vi "WFDC Scan Focus.vi"(0 "Ref Image":T1, 5 "Camera Notifier":string, 7 "Z Stage Notifier":string, 9 "No. of Steps":i32=40, 11 "Step Size (µm)":dbl=1.0) -> (4 "Z Stage Notifier (Dup)":string, 8 "Pos vs. Corr":dbl[][](array[numeric]), 15 "Canceled?":bool)   [LabVIEW 2020]
uses:
  <vilib>/vision/Image Controls.llb/IMAQ Image.ctl
  <vilib>/Utility/miscctls.llb/LVPointTypeDef.ctl
  Device Library/Stages/Stages Controls/Stage Actions.ctl
panel:
  in  "Cancel":bool
  out "Position vs. Normalized Correlation":cluster{dbl[], dbl[]}(graph)
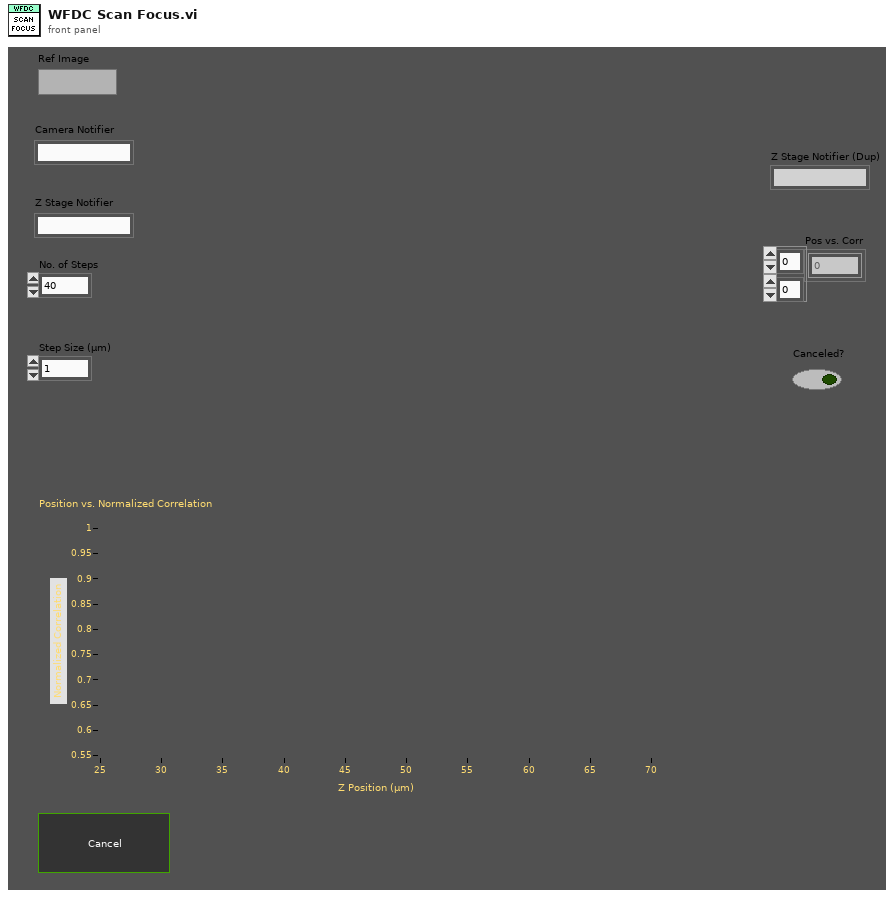
[diagram p1: front panel]
types:
  T1 = typedef "IMAQ Image.ctl" = refnum<image>
  T2 = enum16{"Always On", "Always Off", "Off While Running"}
  T3 = typedef "LVPointTypeDef.ctl" = cluster{"Horizontal":i16, "Vertical":i16}
  T4 = typedef "LVRectTypeDef.ctl" = cluster{"Left":i16, "Top":i16, "Right":i16, "Bottom":i16}
  T5 = typedef "LVBoundsTypeDef.ctl" = cluster{"Width":u32, "Height":u32}
  T6 = typedef "Stage Actions.ctl" = enum16{"Get Position", "MVR", "MOVE", "HALT", "ONTARGET", "ERROR", "REFERENCE", "INIT", "VELOCITY", "STATUS", "EXIT", "HOME", "ZEROPOS", "NANOPOS", "ANALOG", "QUIT"}
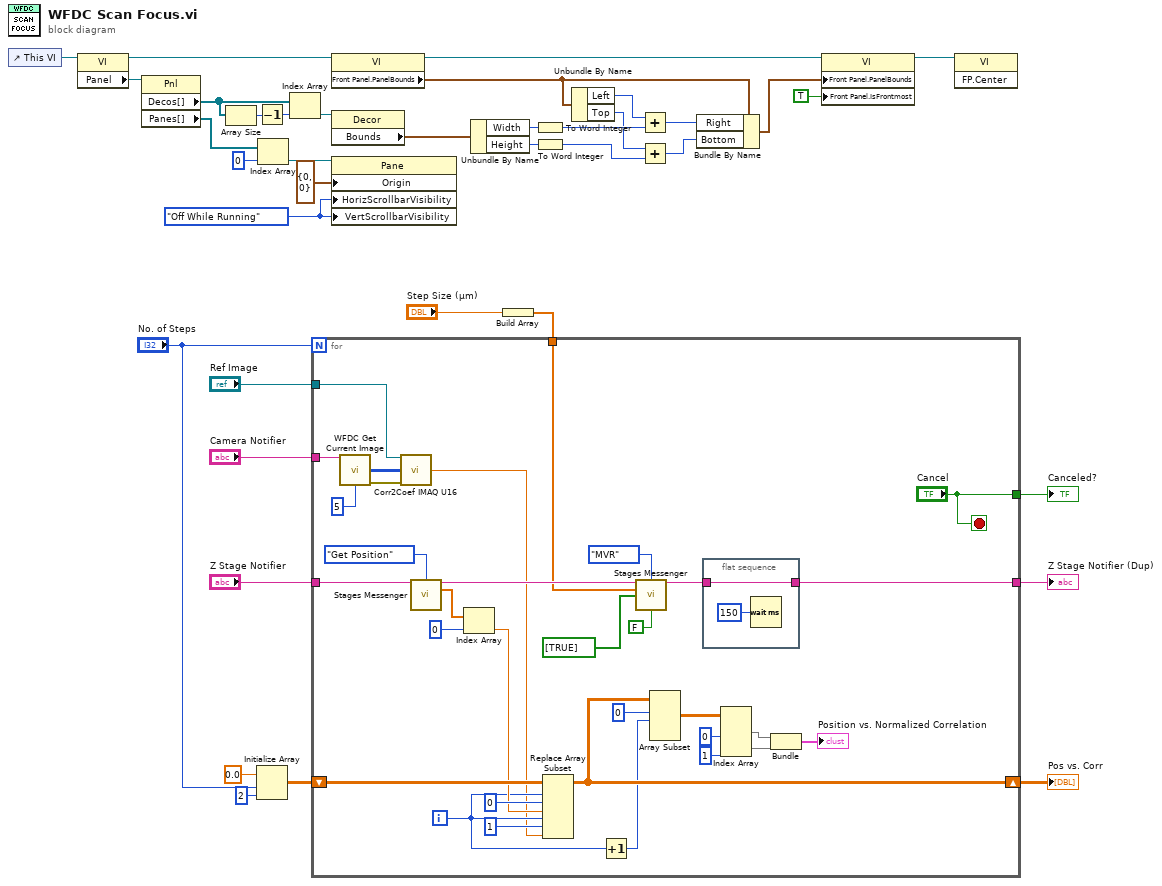
[diagram p0: block diagram]
diagram:
  w16 = T2."Off While Running" ("Vertical Scrollbar Visibility")
  n1 = control-ref of="This VI"() -> (w3:refnum<vi>)
  n2 = property class="VI"(reference=w3) -> (reference out=w17:refnum<vi>, "Panel"=w10:refnum<vi>)  [unwired: 1 in, 1 out]
  n3 = property class="Pnl"(reference=w10) -> ("Decos[]"=w9:refnum<vi>[], "Panes[]"=w13:refnum<vi>[])  [unwired: 1 in, 2 out]
  n4 = Array Size(array=w9) -> (size(s)=w7:i32)
  n5 = Decrement(x=w7) -> (x-1=w8:i32)
  n6 = Initialize Array(0.0 ("element"), "No. of Steps", 2 ("dimension size")) -> (w37:dbl[][])
  n7 = Index Array(array=w13, index=0) -> (element=w12:refnum<vi>)
  n8 = Index Array(array=w9, index=w8) -> (element=w15:refnum<vi>)
  n9 = property class="VI"(reference=w17) -> (reference out=w19:refnum<vi>, "Front Panel.PanelBounds"=w20:T4)  [unwired: 1 in, 1 out]
  n10 = property class="Decor"(reference=w15) -> ("Bounds"=w18:T5)  [unwired: 1 in, 2 out]
  n11 = property class="Pane"(reference=w12, "Origin"=T3 {"Horizontal"=0, "Vertical"=0}, "HorizScrollbarVisibility"=w16, "VertScrollbarVisibility"=w16) -> ()  [unwired: 1 in, 2 out]
  n12 = Unbundle By Name(w18) -> ("Width"=w23:u32, "Height"=w26:u32)
  n13 = Build Array("Step Size (µm)") -> (w29:dbl[])
  n14 = for {
    N: "No. of Steps" -> [_]
    tunnel: "Camera Notifier" -> [w69]
    tunnel: "Z Stage Notifier" -> [w65]
    tunnel: "Ref Image" -> [w40]
    shift-right: [w52] -> w31
    shift-left: w37 -> [w62]
    tunnel: [w43] -> w34
    tunnel: w29 -> [w47]
    tunnel: ["Cancel"] -> w28
    i -> [w49]
    stop <- "Cancel" stop-if-true
    n15 = call "WFDC Get Current Image.vi"("IDS Camera Notifier Name"=w69, "Frames"=u16 5) -> ("Image - U16"=w41:u16[][], "Error"=w42:errorcluster)  [unwired: 11 in, 1 out]
    n16 = call "Corr2Coef IMAQ U16.vi"("Image A"=w40, "Image B"=w41, "Error In"=w42) -> ("Corr Coef"=w39:dbl)  [unwired: 11 in, 1 out]
    n17 = call "Stages Messenger.vi"("Stage Notifier Name"=w65, "Actions"=Stage_Actions."Get Position") -> ("Stage Notifier Name (Dup)"=w59:string, "Positions"=w64:dbl[])  [unwired: 9 in, 3 out]
    n18 = Index Array(array=w64, index=0) -> (element=w57:dbl)
    n19 = Replace Array Subset(array=w62, new element #1=w57, index (row) #1=w49, index (col) #1=0 ("disabled index (col)"), new element #2=w39, index (row) #2=w49, index (col) #2=1 ("disabled index (col)")) -> (w52:dbl[][])
    n20 = Increment(x=w49) -> (x+1=w48:i32)
    n21 = call "Stages Messenger.vi"("Stage Notifier Name"=w59, "Actions"=Stage_Actions."MVR", "Setpoint"=w47, "Axis"=bool[] [TRUE], "Exit While Busy?"=FALSE) -> ("Stage Notifier Name (Dup)"=w44:string)  [unwired: 6 in, 4 out]
    n22 = Array Subset(array=w52, index (row)=0 ("index"), length (row)=w48) -> (w51:dbl[][])  [unwired: 2 in]
    n23 = flat-sequence {
      tunnel: w44 -> [w72]
      tunnel: [w72] -> w43
      frame #0 {
        n24 = Wait (ms)(milliseconds to wait=u32 150) -> ()  [unwired: 1 out]
      }
    }
    n25 = Index Array(array=w51, index (col) #1=0 ("disabled index (col)"), index (col) #2=1 ("index (col)")) -> (element #1=w54:dbl[], element #2=w53:dbl[])  [unwired: 2 in]
    n26 = Bundle(w54, w53) -> (→"Position vs. Normalized Correlation":cluster{dbl[], dbl[]})  [unwired: 1 in]
  }
  "Z Stage Notifier (Dup)" <- w34
  "Pos vs. Corr" <- w31
  "Canceled?" <- w28
  n27 = To Word Integer(number=w23) -> (16bit integer=w25:i16)
  n28 = To Word Integer(number=w26) -> (16bit integer=w4:i16)
  n29 = Unbundle By Name(w20) -> ("Left"=w22:i16, "Top"=w6:i16)
  n30 = Add(x=w22, y=w25) -> (x+y=w24:i16)
  n31 = Add(x=w6, y=w4) -> (x+y=w5:i16)
  n32 = Bundle By Name(cluster=w20, "Right"=w24, "Bottom"=w5) -> (w21:T4)
  n33 = property class="VI"(reference=w19, "Front Panel.PanelBounds"=w21, "Front Panel.IsFrontmost"=TRUE ("Front Panel Window:Is Frontmost")) -> (reference out=w1:refnum<vi>)  [unwired: 1 in, 1 out]
  n34 = invoke class="VI" method="FP.Center"(reference=w1) -> ()  [unwired: 2 in, 3 out]
